vi "ErrorHandler.vi"(6 "EnqueueType (QMH)":T1, 8 "error in (no error)":errorcluster, 11 "Queue Names":string[](array[string])) -> (0 "error out":errorcluster)   [LabVIEW 2018, in "AcPwrPlugins.lvlib"]
doc: "This VI checks if an error occurs. If so it puts the error contents into the messaging queue to be handled in detail later."
uses:
  AcPwrPlugins.lvlib
  QueueTypeEnum.ctl
  EnqueueEnum.ctl
panel:
  in  "Message (Error)":string="Error"
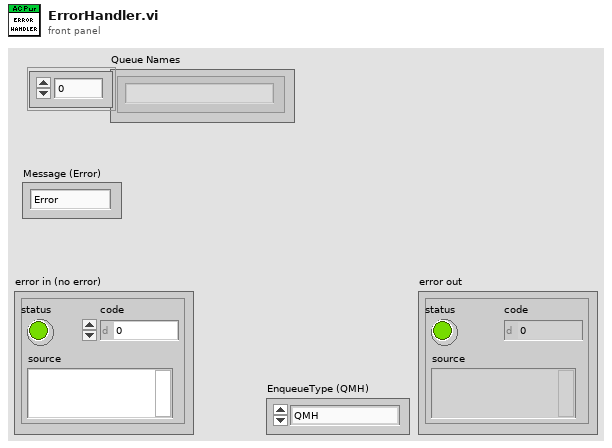
[diagram p1: front panel]
types:
  T1 = typedef "AcPwrPlugins.lvlib/QueueTypeEnum.ctl" = enum16{"QMH", "Class ", "MA"}
  T2 = typedef "AcPwrPlugins.lvlib/EnqueueEnum.ctl" = enum16{"LossyEnqueue", "EnqueueAtFront", "Enqueue"}
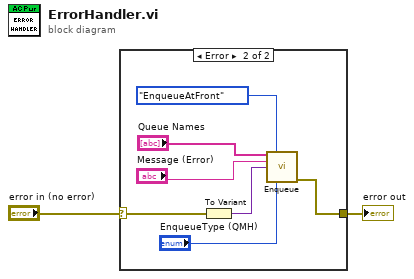
[diagram p0: block diagram]
diagram:
  n1 = case shown="Error" "error in (no error)" {
    selector: "error in (no error)" -> [w3 w10]
    tunnel: [w3 w8] -> w1
    frame No Error {
    }
    frame Error {
      n2 = To Variant(anything=w10) -> (Variant=w9:variant)
      n3 = call "Enqueue.vi"("Queue Names"="Queue Names", "EnqueueType (Enqueue)"=EnqueueEnum."EnqueueAtFront", "Message"="Message (Error)", "Message Data"=w9, "EnqueueType (QMH)"="EnqueueType (QMH)") -> ("error out"=w8:errorcluster)  [unwired: 9 in, 1 out]
    }
  }
  "error out" <- w1
